vi "Query Frame Insert&Update.vi"(4 "Where Data":string, 6 "Action":T1, 7 "Where Condition":string, 8 "FP Data":string[](array[string]), 9 "DB Column Name":string[](array[string]), 10 "Table Name":string, 11 "Schema":string) -> (3 "Query":string)   [LabVIEW 2023, in "HardwareAbstractionLayer_LVOOP.lvlib" / "MYSQL Database.lvclass"]
uses:
  MYSQL Database.lvclass
  Control/Query Action.ctl
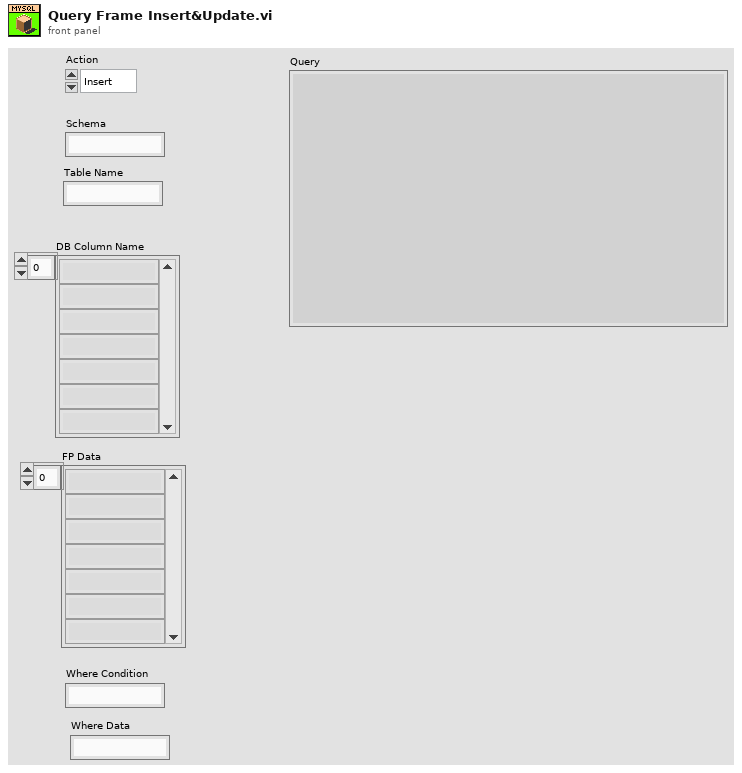
[diagram p1: front panel]
types:
  T1 = typedef "HardwareAbstractionLayer_LVOOP.lvlib/MYSQL Database.lvclass/Query Action.ctl" = enum16{"Insert", "Update"}
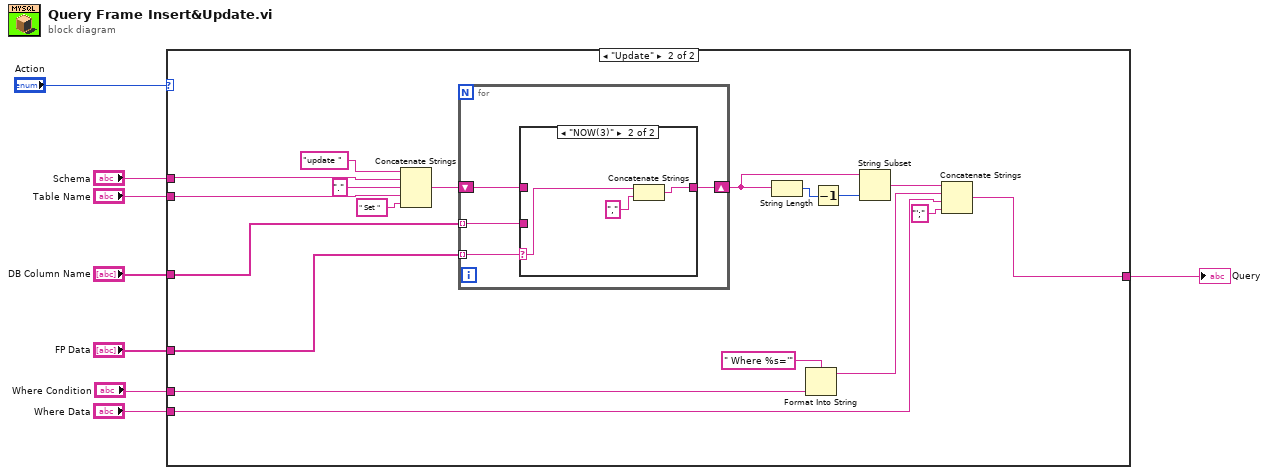
[diagram p0: block diagram]
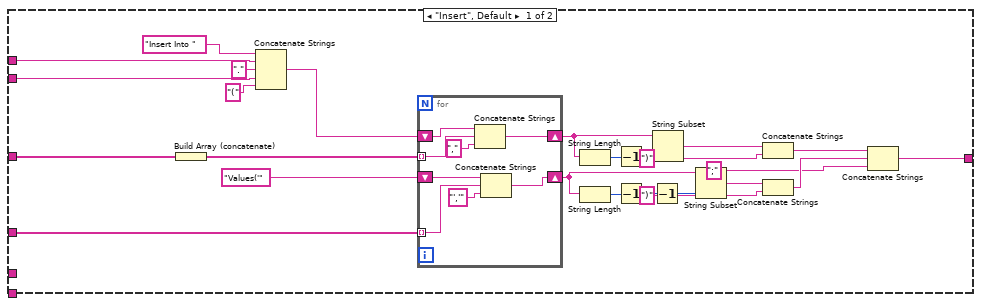
[diagram p2: hidden frame]
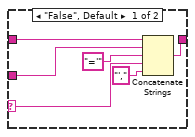
[diagram p3: hidden frame]
diagram:
  n1 = case shown="\"Update\"" "Action" {
    tunnel: "DB Column Name" -> [w33 w48]
    tunnel: "FP Data" -> [w32 w47]
    tunnel: "Table Name" -> [w31 w49]
    tunnel: "Schema" -> [w29 w50]
    tunnel: [w28 w42] -> w4
    tunnel: "Where Data" -> [_ w46]
    tunnel: "Where Condition" -> [_ w43]
    frame "Insert", Default {
      n2 = Build Array (concatenate)(w33) -> (w30:string[])
      n3 = Concatenate Strings("Insert Into " ("string"), w29, "." ("string"), w31, "(" ("string")) -> (w26:string)
      n4 = for {
        shift-right: [w38] -> w22
        shift-left: w26 -> [w41]
        tunnel: w30 -> [w40] mode=indexing
        shift-right: [w34] -> w18
        shift-left: "Values('" -> [w37]
        tunnel: w32 -> [w36] mode=indexing
        n5 = Concatenate Strings(w41, w40, "," ("string")) -> (w38:string)
        n6 = Concatenate Strings(w37, w36, "','" ("string")) -> (w34:string)
      }
      n7 = String Length(string=w22) -> (length=w24:i32)
      n8 = String Length(string=w18) -> (length=w21:i32)
      n9 = Decrement(x=w24) -> (x-1=w23:i32)
      n10 = Decrement(x=w21) -> (x-1=w20:i32)
      n11 = Decrement(x=w20) -> (x-1=w19:i32)
      n12 = String Subset(string=w22, length (rest)=w23) -> (substring=w17:string)  [unwired: 1 in]
      n13 = String Subset(string=w18, length (rest)=w19) -> (substring=w15:string)  [unwired: 1 in]
      n14 = Concatenate Strings(w17, ")" ("string")) -> (w13:string)
      n15 = Concatenate Strings(w15, ")" ("string")) -> (w12:string)
      n16 = Concatenate Strings(w13, w12, ";" ("string")) -> (w28:string)
    }
    frame "Update" {
      n17 = Concatenate Strings("update " ("string"), w50, "." ("string"), w49, " Set " ("string")) -> (w58:string)
      n18 = for {
        shift-right: [w62] -> w55
        shift-left: w58 -> [w63]
        tunnel: w48 -> [w61] mode=indexing
        tunnel: w47 -> [w60] mode=indexing
        n19 = case shown="\"NOW(3)\"" w60 {
          selector: w60 -> [w65 w72]
          tunnel: w63 -> [w69 _]
          tunnel: [w68 w71] -> w62
          tunnel: w61 -> [w67 _]
          frame "False", Default {
            n20 = Concatenate Strings(w69, w67, "='" ("string"), w65, "'," ("string")) -> (w68:string)
          }
          frame "NOW(3)" {
            n21 = Concatenate Strings(w72, "," ("string")) -> (w71:string)
          }
        }
      }
      n22 = String Length(string=w55) -> (length=w57:i32)
      n23 = Format Into String(format string=" Where %s='" ("string"), w43) -> (resulting string=w44:string)  [unwired: 2 in, 1 out]
      n24 = Decrement(x=w57) -> (x-1=w56:i32)
      n25 = String Subset(string=w55, length (rest)=w56) -> (substring=w52:string)  [unwired: 1 in]
      n26 = Concatenate Strings(w52, w44, w46, "';" ("string")) -> (w42:string)
    }
  }
  "Query" <- w4
